vi "Field Draw Path.vi"(0 "Pontos Smooth":dbl[][](array[numeric]), 1 "function":T1=enum."Attacker", 4 "Lado":enum16{"Esquerdo", "Direito"}(ring) caption="Enum", 6 "Draw Targets?":T3, 8 "Scale mm/pixel":dbl, 9 "Offset":T4, 10 "Pontos":dbl[][](array[numeric]), 11 "picture in":picture) -> (2 "picture out":picture)   [LabVIEW 2023]
uses:
  <vilib>/Utility/miscctls.llb/LVBoundsTypeDef.ctl
  DrawTargets.ctl
  Controls/Functions Enum.ctl
panel:
  in  "pen 2":T2={"Width"=3, "Style"=enum."Solid"}
  in  "pen":T2={"Width"=3, "Style"=enum."Solid"}
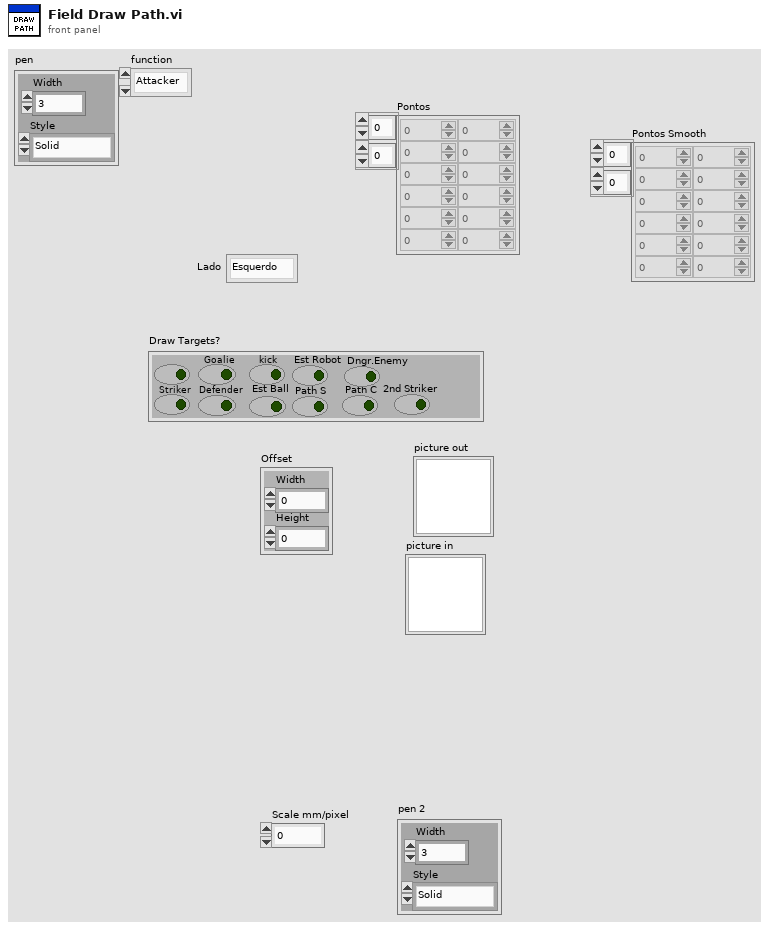
[diagram p1: front panel]
types:
  T1 = typedef "Functions Enum.ctl" = enum16{"2nd Striker", "Attacker", "Goalie", "Defender", "Striker", "Goto 0", "Dummy", "Kicker", "ZigZag 0", "ZigZag 1", "ZigZag 2", "ZigZag 3", "ZigZag 4", "ZigZag 5", "ZigZag 6", "ZigZag 7", "ZigZag 8", ""}
  T2 = cluster{"Width":u16, "Style":enum32{"Solid", "Dash", "Dot", "DashDot", "DashDotDot"}}
  T3 = typedef "DrawTargets.ctl" = cluster{"Attacker":bool, "Striker":bool, "Goalie":bool, "Defender":bool, "kick":bool, "Est Ball":bool, "Est Robot":bool, "Path S":bool, "Path C":bool, "Dngr.Enemy":bool, "2nd Striker":bool}
  T4 = typedef "LVBoundsTypeDef.ctl" = cluster{"Width":u32, "Height":u32}
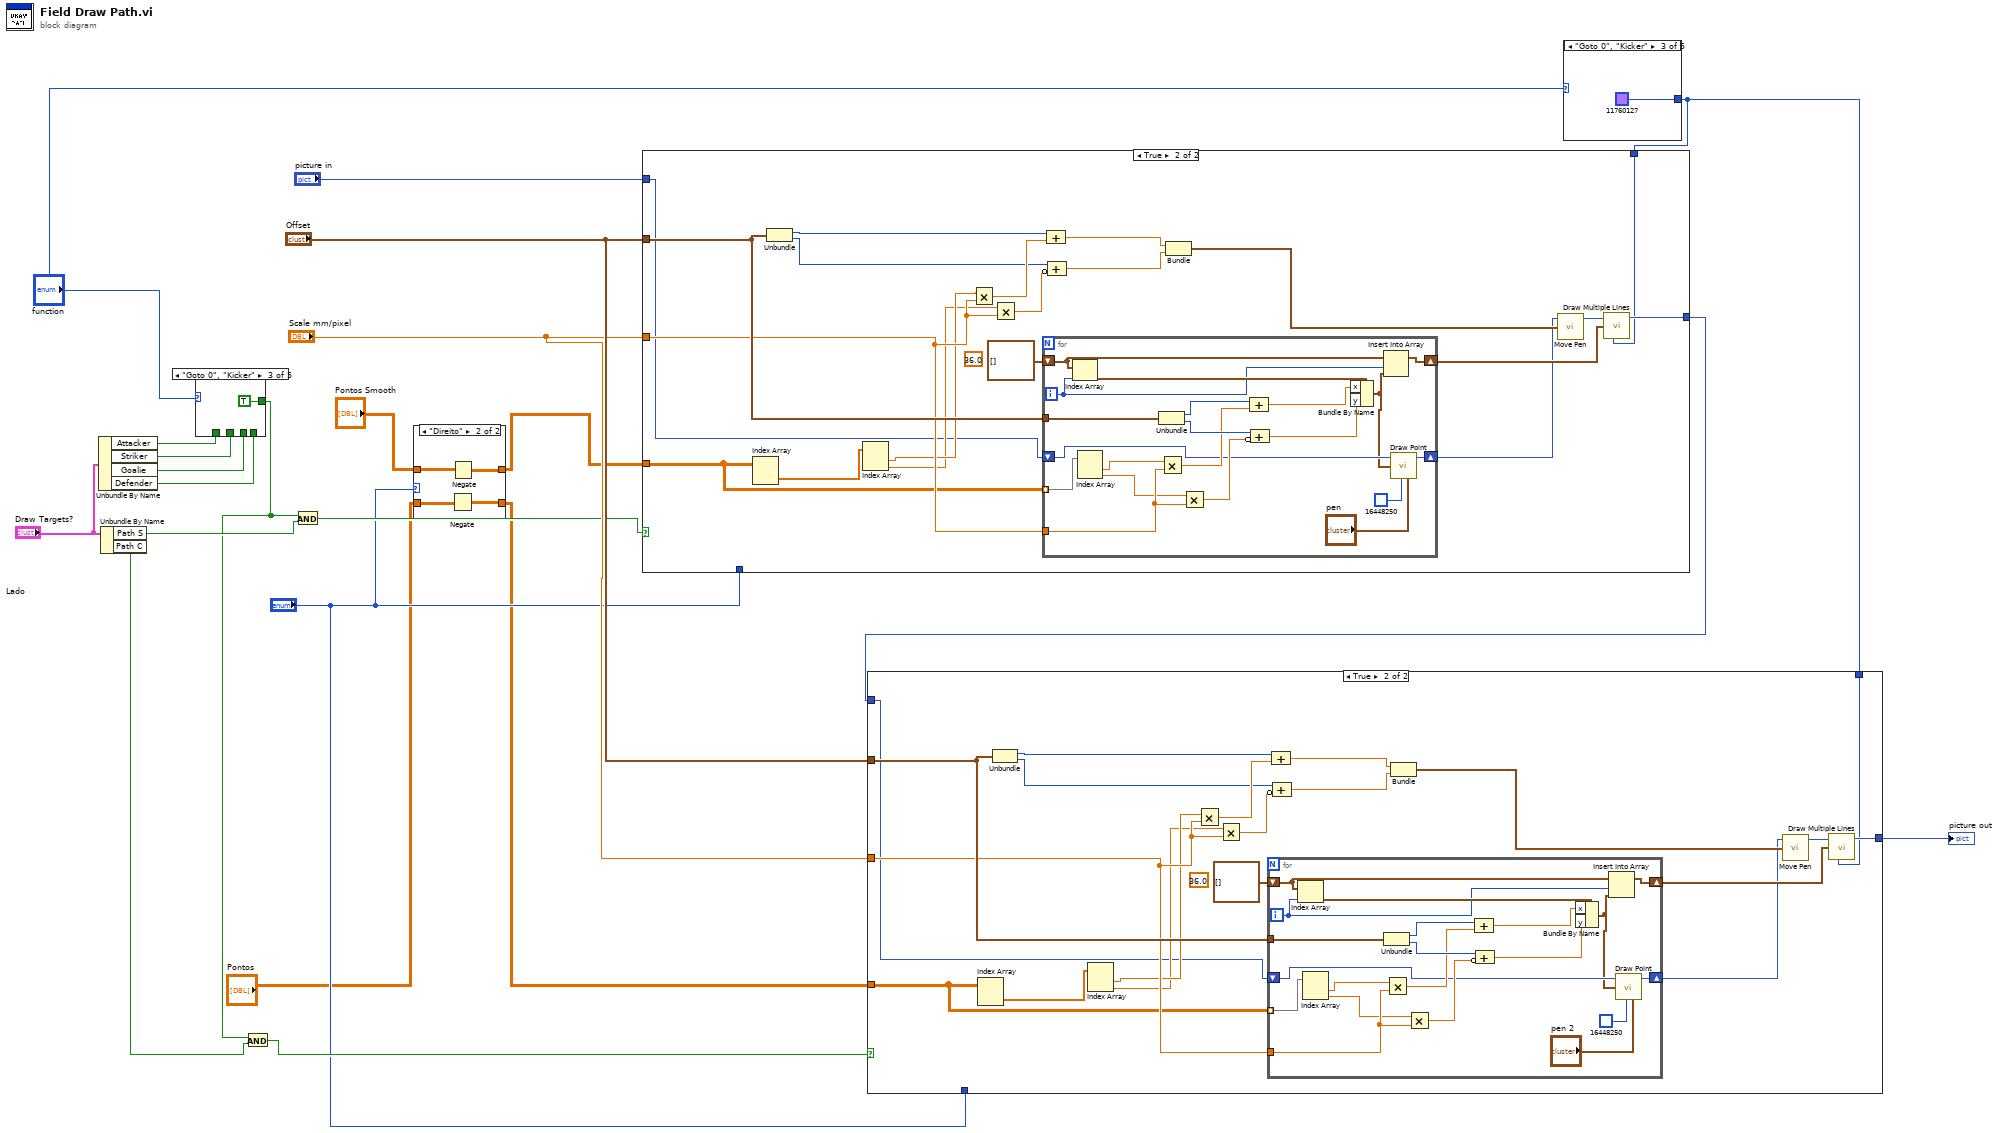
[diagram p0: block diagram]
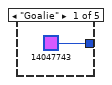
[diagram p7: hidden frame]
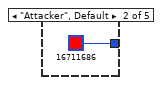
[diagram p8: hidden frame]
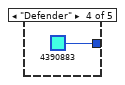
[diagram p9: hidden frame]
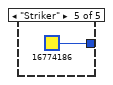
[diagram p10: hidden frame]
diagram:
  n1 = Unbundle By Name("Draw Targets?") -> ("Attacker"=w14:bool, "Striker"=w15:bool, "Goalie"=w13:bool, "Defender"=w16:bool)
  n2 = Unbundle By Name("Draw Targets?") -> ("Path S"=w9:bool, "Path C"=w7:bool)
  n3 = case shown="\"Goto 0\", \"Kicker\"" "function" {
    tunnel: [w23 w24 TRUE ("Draw Target Striker?") w26 w27] -> w8
    tunnel: w16 -> [_ _ _ w26 _]
    tunnel: w15 -> [_ _ _ _ w27]
    tunnel: w14 -> [w23 _ _ _ _]
    tunnel: w13 -> [_ w24 _ _ _]
    frame "Attacker", Default {
    }
    frame "Goalie" {
    }
    frame "Goto 0", "Kicker" {
    }
    frame "Defender" {
    }
    frame "Striker" {
    }
  }
  n4 = And(x=w8, y=w7) -> (x .and. y?=w6:bool)
  n5 = And(x=w8, y=w9) -> (x .and. y?=w10:bool)
  n6 = case shown="\"Direito\"" "Lado" {
    tunnel: "Pontos Smooth" -> [w29 w31]
    tunnel: [w29 w30] -> w3
    tunnel: "Pontos" -> [w28 w33]
    tunnel: [w28 w32] -> w1
    frame "Esquerdo", Default {
    }
    frame "Direito" {
      n7 = Negate(x=w33) -> (-x=w32:dbl[][])
      n8 = Negate(x=w31) -> (-x=w30:dbl[][])
    }
  }
  n9 = case shown="\"Goto 0\", \"Kicker\"" "function" {
    tunnel: [u32 14047743 ("color(black)") u32 16711686 ("color(black)") u32 11760127 ("color(black)") u32 4390883 ("color(black)") u32 16774186 ("color(black)")] -> w17
    frame "Goalie" {
    }
    frame "Attacker", Default {
    }
    frame "Goto 0", "Kicker" {
    }
    frame "Defender" {
    }
    frame "Striker" {
    }
  }
  n10 = case shown="True" w10 {
    tunnel: [w39 w41] -> w21
    tunnel: "Offset" -> [_ w52]
    tunnel: "Scale mm/pixel" -> [_ w51]
    tunnel: "picture in" -> [w39 w43]
    tunnel: "Lado" -> [_ _]
    tunnel: w3 -> [_ w46]
    tunnel: w17 -> [_ w40]
    frame False {
    }
    frame True {
      (unwired) sgl 36.0 ("radius")
      n11 = Index Array(array=w46) -> (element=w49:dbl[])  [unwired: 2 in]
      n12 = Unbundle(w52) -> ("Width"=w59:u32, "Height"=w56:u32)
      n13 = Index Array(array=w49) -> (element #1=w48:dbl, element #2=w47:dbl)  [unwired: 2 in]
      n14 = Multiply(x=w48, y=w51) -> (x*y=w58:dbl)
      n15 = Multiply(x=w47, y=w51) -> (x*y=w55:dbl)
      n16 = for {
        tunnel: w52 -> [w77]
        tunnel: w51 -> [w76]
        tunnel: w46 -> [w73] mode=indexing
        shift-right: [w65] -> w44
        shift-left: cluster{"x":i16, "y":i16}[] [] ("line endpoints") -> [w66]
        shift-right: [w63] -> w42
        shift-left: w43 -> [w64]
        i -> [w67]
        n17 = Index Array(array=w66, index=w67) -> (element=w68:cluster{"x":i16, "y":i16})
        n18 = Index Array(array=w73) -> (element #1=w72:dbl, element #2=w71:dbl)  [unwired: 2 in]
        n19 = Unbundle(w77) -> ("Width"=w79:u32, "Height"=w78:u32)
        n20 = Multiply(x=w72, y=w76) -> (x*y=w75:dbl)
        n21 = Multiply(x=w71, y=w76) -> (x*y=w74:dbl)
        n22 = Compound Arithmetic op=ADD(w79, w75) -> (w70:dbl)
        n23 = Compound Arithmetic op=ADD(w78, invert w74) -> (w69:dbl)
        n24 = Bundle By Name(cluster=w68, "x"=w70, "y"=w69) -> (w61:cluster{"x":i16, "y":i16})
        n25 = Insert Into Array(array=w66, index=w67, new element=w61) -> (w65:cluster{"x":i16, "y":i16}[])
        n26 = call <vilib>:"Draw Point.vi"("picture"=w64, "point(x,y)"=w61, "color(black)"=u32 16448250, "pen"="pen") -> ("new picture"=w63:picture)  [unwired: 5 in]
      }
      n27 = Compound Arithmetic op=ADD(w59, w58) -> (w57:dbl)
      n28 = Compound Arithmetic op=ADD(w56, invert w55) -> (w54:dbl)
      n29 = Bundle(w57, w54) -> (w50:cluster{dbl, dbl})  [unwired: 1 in]
      n30 = call <vilib>:"Move Pen.vi"("new position"=w50, "picture"=w42) -> ("new picture"=w53:picture)  [unwired: 3 in]
      n31 = call <vilib>:"Draw Multiple Lines.vi"("picture"=w53, "line endpoints"=w44, "color(black)"=w40) -> ("new picture"=w41:picture)  [unwired: 6 in]
    }
  }
  n32 = case shown="True" w6 {
    tunnel: [w80 w82] -> w18
    tunnel: "Offset" -> [_ w93]
    tunnel: "Scale mm/pixel" -> [_ w92]
    tunnel: w21 -> [w80 w84]
    tunnel: "Lado" -> [_ _]
    tunnel: w1 -> [_ w87]
    tunnel: w17 -> [_ w81]
    frame False {
    }
    frame True {
      (unwired) sgl 36.0 ("radius")
      n33 = Index Array(array=w87) -> (element=w90:dbl[])  [unwired: 2 in]
      n34 = Unbundle(w93) -> ("Width"=w100:u32, "Height"=w97:u32)
      n35 = Index Array(array=w90) -> (element #1=w89:dbl, element #2=w88:dbl)  [unwired: 2 in]
      n36 = Multiply(x=w89, y=w92) -> (x*y=w99:dbl)
      n37 = Multiply(x=w88, y=w92) -> (x*y=w96:dbl)
      n38 = for {
        tunnel: w93 -> [w118]
        tunnel: w92 -> [w117]
        tunnel: w87 -> [w114] mode=indexing
        shift-right: [w106] -> w85
        shift-left: cluster{"x":i16, "y":i16}[] [] ("line endpoints") -> [w107]
        shift-right: [w104] -> w83
        shift-left: w84 -> [w105]
        i -> [w108]
        n39 = Index Array(array=w107, index=w108) -> (element=w109:cluster{"x":i16, "y":i16})
        n40 = Index Array(array=w114) -> (element #1=w113:dbl, element #2=w112:dbl)  [unwired: 2 in]
        n41 = Unbundle(w118) -> ("Width"=w120:u32, "Height"=w119:u32)
        n42 = Multiply(x=w113, y=w117) -> (x*y=w116:dbl)
        n43 = Multiply(x=w112, y=w117) -> (x*y=w115:dbl)
        n44 = Compound Arithmetic op=ADD(w120, w116) -> (w111:dbl)
        n45 = Compound Arithmetic op=ADD(w119, invert w115) -> (w110:dbl)
        n46 = Bundle By Name(cluster=w109, "x"=w111, "y"=w110) -> (w102:cluster{"x":i16, "y":i16})
        n47 = Insert Into Array(array=w107, index=w108, new element=w102) -> (w106:cluster{"x":i16, "y":i16}[])
        n48 = call <vilib>:"Draw Point.vi"("picture"=w105, "point(x,y)"=w102, "color(black)"=u32 16448250, "pen"="pen 2") -> ("new picture"=w104:picture)  [unwired: 5 in]
      }
      n49 = Compound Arithmetic op=ADD(w100, w99) -> (w98:dbl)
      n50 = Compound Arithmetic op=ADD(w97, invert w96) -> (w95:dbl)
      n51 = Bundle(w98, w95) -> (w91:cluster{dbl, dbl})  [unwired: 1 in]
      n52 = call <vilib>:"Move Pen.vi"("new position"=w91, "picture"=w83) -> ("new picture"=w94:picture)  [unwired: 3 in]
      n53 = call <vilib>:"Draw Multiple Lines.vi"("picture"=w94, "line endpoints"=w85, "color(black)"=w81) -> ("new picture"=w82:picture)  [unwired: 6 in]
    }
  }
  "picture out" <- w18
